vi "ILMMonitor.vi"() -> ()   [LabVIEW 2015]
uses:
  Oxford Software/Oxsoft/BUSGEN.LLB/OxfordAddress.ctl
  Global/Global Variables/Data_Display_global.vi
panel:
  out "Nitrogen Level":dbl format="%#4_5f"
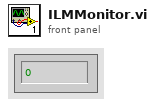
[diagram p1: front panel]
types:
  T1 = typedef "OxfordAddress.ctl" = cluster{"Com Port":i32, "ISOBUS Address":i32, "GPIB Address":i16, "Communication":enum16{"RS232", "ISOBUS", "GPIB", "Gateway"}}
  T2 = typedef "ILMChannelStatus.ctl" = cluster{"Probe current":bool, "Probe fast":bool, "Probe slow":bool, "Auto-fill":enum16{"End fill", "Not filling", "Filling", "Start filling"}, "Fill":bool, "Low level":bool, "Alm requested":bool, "Pre-pulse I":bool}
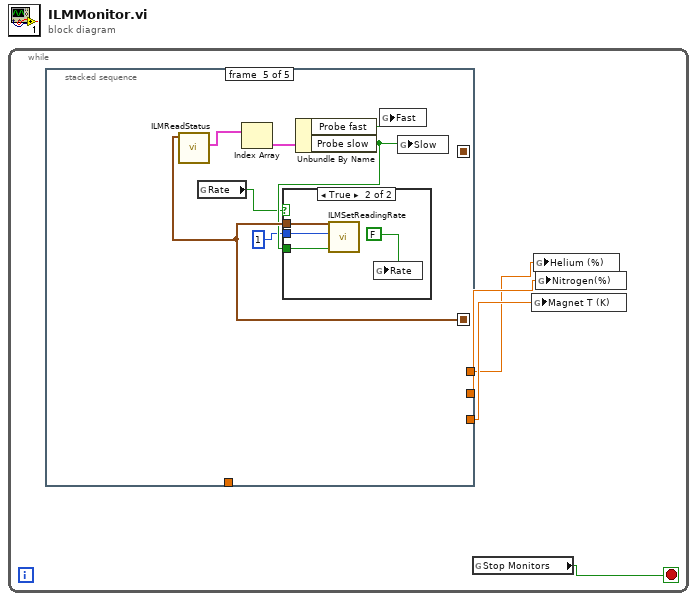
[diagram p0: block diagram]
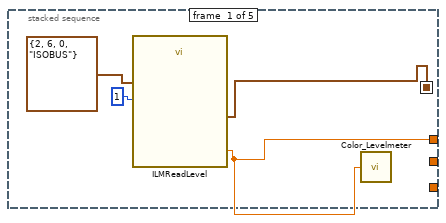
[diagram p2: hidden frame]
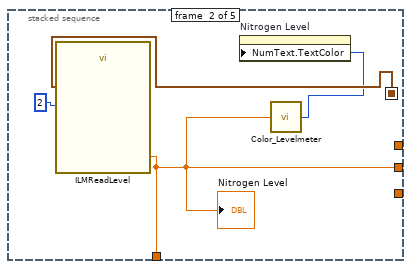
[diagram p3: hidden frame]
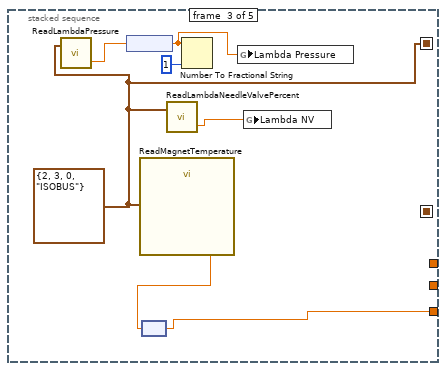
[diagram p4: hidden frame]
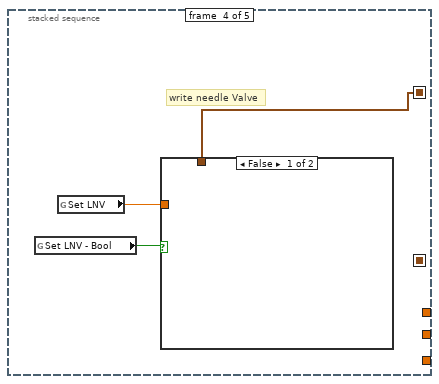
[diagram p5: hidden frame]
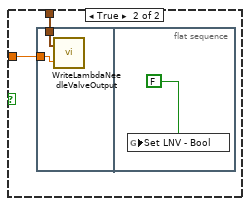
[diagram p6: hidden frame]
diagram:
  n1 = while {
    stop <- w4 stop-if-true
    n2 = stacked-sequence {
      seq-local: [w6 _ _ _ _] -> [_ w11 _ _ w34]
      seq-local: [_ _ w15 _ _] -> [_ _ _ w22 _]
      tunnel: [_ w9 _ _ _] -> _
      tunnel: [_ _ w18 _ _] -> w3
      tunnel: [_ w9 _ _ _] -> w2
      tunnel: [w5 _ _ _ _] -> w1
      frame #0 {
        n3 = call "ILMReadLevel.vi"("Address"=T1 {"Com Port"=2, "ISOBUS Address"=6, "GPIB Address"=0, "Communication"=enum."ISOBUS"}, "Channel number (1-3)"=u8 1) -> ("Address(thru)"=w6:T1, "Level"=w5:dbl)  [unwired: 1 out]
        n4 = call "Color_Levelmeter.vi"("In"=w5) -> ()  [unwired: 1 out]
      }
      frame #1 {
        n5 = call "ILMReadLevel.vi"("Address"=w11, "Channel number (1-3)"=u8 2) -> ("Level"=w9:dbl)  [unwired: 2 out]
        "Nitrogen Level" <- w9
        n6 = call "Color_Levelmeter.vi"("In"=w9) -> ("Out"=w10:i32)
        n7 = property on="Nitrogen Level" class="DigNum (strict)"("NumText.TextColor"=w10) -> ()  [unwired: 2 in, 2 out]
      }
      frame #2 {
        w15 = T1 {"Com Port"=2, "ISOBUS Address"=3, "GPIB Address"=0, "Communication"=enum."ISOBUS"} ("Address")
        n8 = call "ReadLambdaPressure.vi"("Address"=w15) -> ("Pressure"=w16:dbl[unit])  [unwired: 1 in, 1 out]
        n9 = node(w16) -> (w13:dbl)
        n10 = call "ReadMagnetTemperature.vi"("Address"=w15) -> ("Magnet Temperature"=w19:dbl[unit])  [unwired: 1 in, 1 out]
        n11 = node(w19) -> (w18:dbl)
        n12 = call "ReadLambdaNeedleValvePercent.vi"("Address"=w15) -> ("Actual Needle Valve  %"=w14:dbl)  [unwired: 1 in, 1 out]
        n13 = Number To Fractional String(number=w13, precision (6)=1) -> ()  [unwired: 2 in, 1 out]
        n14 = global write "Data_Display_global.vi" "Lambda Pressure"(w13) -> ()
        n15 = global write "Data_Display_global.vi" "Lambda NV"(w14) -> ()
      }
      frame #3 {
        # "write needle Valve"
        n16 = global read "Data_Display_global.vi" "Set LNV - Bool"() -> (w20:bool)
        n17 = global read "Data_Display_global.vi" "Set LNV"() -> (w21:dbl)
        n18 = case shown="False" w20 {
          tunnel: w22 -> [_ w24]
          tunnel: w21 -> [_ w23]
          frame False {
          }
          frame True {
            n19 = flat-sequence {
              tunnel: w24 -> [w26]
              tunnel: w23 -> [w25]
              frame #0 {
                n20 = call "WriteLambdaNeedleValveOutput.vi"("Needle Valve Output (%)"=w25, "Address"=w26) -> ()  [unwired: 1 in, 1 out]
              }
              frame #1 {
                n21 = global write "Data_Display_global.vi" "Set LNV - Bool"(FALSE) -> ()
              }
            }
          }
        }
      }
      frame #4 {
        n22 = call "ILMReadStatus.vi"("Instrument address"=w34) -> ("Channel"=w33:T2[])  [unwired: 3 in, 3 out]
        n23 = global read "Data_Display_global.vi" "Rate"() -> (w28:bool)
        n24 = Index Array(array=w33) -> (element=w32:T2)  [unwired: 1 in]
        n25 = Unbundle By Name(w32) -> ("Probe fast"=w31:bool, "Probe slow"=w30:bool)
        n26 = case shown="True" w28 {
          tunnel: w30 -> [_ w38]
          tunnel: w34 -> [_ w37]
          tunnel: 1 -> [_ w36]
          frame False {
          }
          frame True {
            n27 = call "ILMSetReadingRate.vi"("Fast"=w38, "Channel(1-3)"=w36, "Address"=w37) -> ()  [unwired: 1 out]
            n28 = global write "Data_Display_global.vi" "Rate"(FALSE) -> ()
          }
        }
        n29 = global write "Data_Display_global.vi" "Fast"(w31) -> ()
        n30 = global write "Data_Display_global.vi" "Slow"(w30) -> ()
      }
    }
    n31 = global read "Data_Display_global.vi" "Stop Monitors"() -> (w4:bool)
    n32 = global write "Data_Display_global.vi" "Magnet T (K)"(w3) -> ()
    n33 = global write "Data_Display_global.vi" "Helium (%)"(w1) -> ()
    n34 = global write "Data_Display_global.vi" "Nitrogen(%)"(w2) -> ()
  }
